vi "_testMain.vi"   [LabVIEW 2014]
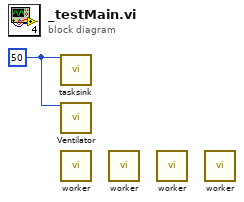
[diagram p0: block diagram]
diagram:
  w1 = 50 ("task_nbr")
  n1 = call "tasksink.vi"("task_nbr"=w1) -> ()  [unwired: 19 in]
  n2 = call "Ventilator.vi"("task_num"=w1) -> ()  [unwired: 19 in]
  n3 = call "worker.vi"() -> ()  [unwired: 20 in]
  n4 = call "worker.vi"() -> ()  [unwired: 20 in]
  n5 = call "worker.vi"() -> ()  [unwired: 20 in]
  n6 = call "worker.vi"() -> ()  [unwired: 20 in]
